vi "SHA-1.vi"(10 "Data":u8[](array[numeric]) format="%02x") -> (2 "message-digest":u8[](array[numeric]) format="%02x")   [LabVIEW 2013, in "SHA-1.lvlib"]
uses:
  SHA-1.lvlib
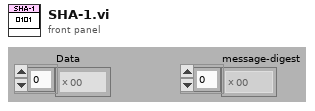
[diagram p1: front panel]
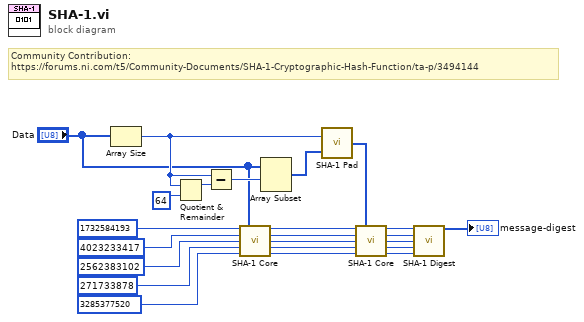
[diagram p0: block diagram]
diagram:
  # "Community Contribution:\nhttps://forums.ni.com/t5/Community-Documents/SHA-1-Cryptographic-Hash-Function/ta-p/3494144"
  n1 = Array Size(array="Data") -> (size(s)=w20:i32)
  n2 = Quotient & Remainder(x=w20, y=64) -> (x-y*floor(x/y)=w22:i32)  [unwired: 1 out]
  n3 = Subtract(x=w20, y=w22) -> (x-y=w23:i32)
  n4 = call "SHA-1 Core.vi"("s1"=u32 1732584193, "Input Bytes"="Data", "s2"=u32 4023233417, "s3"=u32 2562383102, "s4"=u32 271733878, "s5"=u32 3285377520 ("s4")) -> ("s1 out"=w12:u32, "s2 out"=w11:u32, "s3 out"=w10:u32, "s4 out"=w9:u32, "s5 out"=w8:u32)  [unwired: 5 in]
  n5 = Array Subset(array="Data", index=w23) -> (w19:u8[])  [unwired: 1 in]
  n6 = call "SHA-1 Pad.vi"("Last Part"=w19, "Message Length (bytes)"=w20) -> ("Padding"=w7:u8[])
  n7 = call "SHA-1 Core.vi"("s1"=w12, "Input Bytes"=w7, "s2"=w11, "s3"=w10, "s4"=w9, "s5"=w8) -> ("s1 out"=w6:u32, "s2 out"=w5:u32, "s3 out"=w4:u32, "s4 out"=w3:u32, "s5 out"=w2:u32)  [unwired: 5 in]
  n8 = call "SHA-1 Digest.vi"("s1"=w6, "s2"=w5, "s3"=w4, "s4"=w3, "s5"=w2) -> ("message-digest"=→"message-digest":u8[])  [unwired: 10 in]
